vi "DO Test.vi"() -> ()   [LabVIEW 2018]
uses:
  <vilib>/DAQmx/write.llb/DAQmx Write (Digital 1D Bool NChan 1Samp 1Line).vi
  <vilib>/DAQmx/create/channels.llb/DAQmx Create Channel (DO-Digital Output).vi
  <vilib>/DAQmx/miscellaneous.llb/DAQmx Fill In Error Info.vi
  <resource>/objmgr/daqmx.rc
panel:
  in  "index":i32
  out "Array":tag[](array[tag])
  in  "data 2":bool
  in  "Stop":bool
  out "DO.Lines":tag[](array[tag])
  out "DevNames":tag[](array[tag])
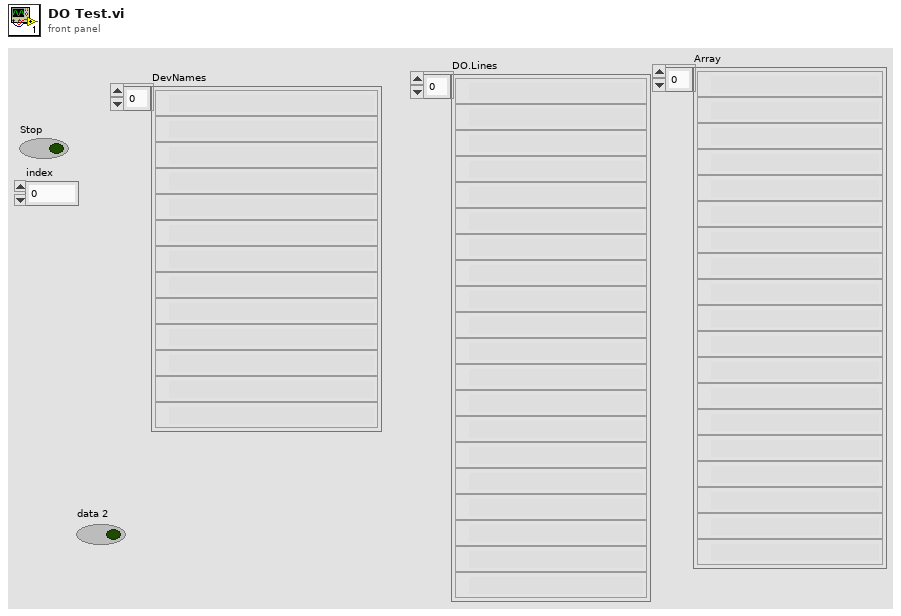
[diagram p1: front panel]
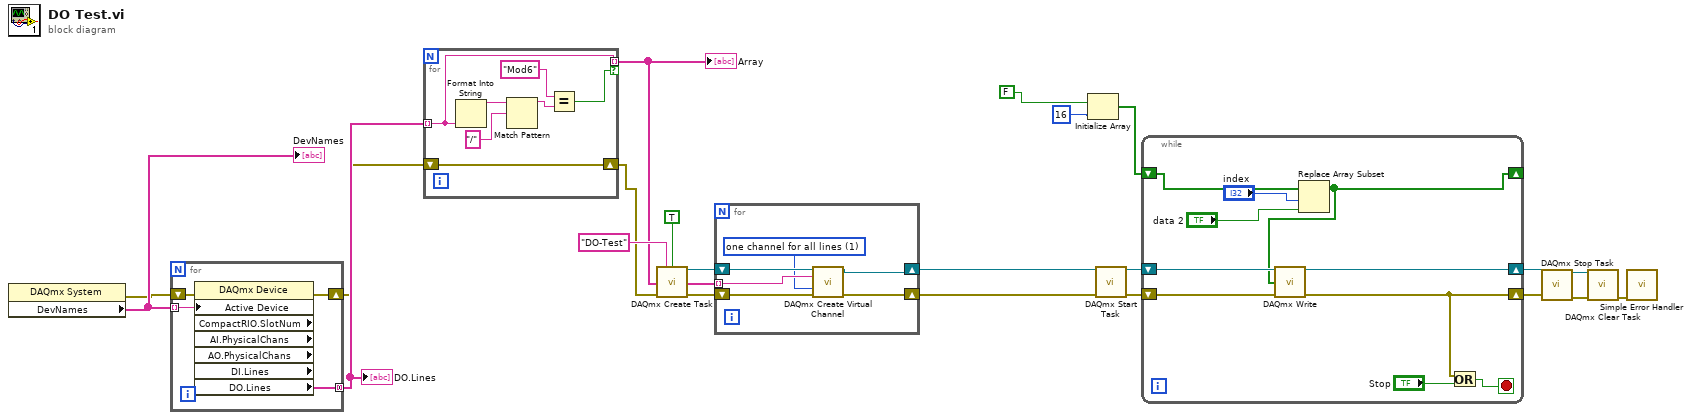
[diagram p0: block diagram]
diagram:
  n1 = property class="DAQmx System"() -> (error out=w17:errorcluster, "DevNames"=w22:tag[])  [unwired: 2 in, 1 out]
  "DevNames" <- w22
  n2 = for {
    tunnel: w22 -> [w26] mode=indexing
    tunnel: [w25] -> w8 mode=concatenating
    shift-right: [w24] -> w6
    shift-left: w17 -> [w23]
    n3 = property class="DAQmx Device" props=["Active Device", "CompactRIO.SlotNum", "AI.PhysicalChans", "AO.PhysicalChans", "DI.Lines", "DO.Lines"](error in=w23, "Active Device"=w26) -> (error out=w24:errorcluster, "DO.Lines"=w25:tag[])  [unwired: 1 in, 5 out]
  }
  "DO.Lines" <- w8
  n4 = for {
    tunnel: w8 -> [w29] mode=indexing
    tunnel: [w29] -> w9 mode=indexing if=w28
    shift-right: [w27] -> w7
    shift-left: w6 -> [w27]
    n5 = Format Into String(w29) -> (resulting string=w33:string)  [unwired: 3 in, 1 out]
    n6 = Match Pattern(string=w33, regular expression="/") -> (before substring=w31:string)  [unwired: 1 in, 3 out]
    n7 = Equal?(x="Mod6" ("before substring"), y=w31) -> (x = y?=w28:bool)
  }
  "Array" <- w9
  n8 = call <vilib>:"DAQmx Create Task.vi"("new task name"="DO-Test", "auto cleanup"=TRUE, "error in"=w7) -> ("task out"=w18:refnum<k21>, "error out"=w19:errorcluster)  [unwired: 11 in]
  n9 = for {
    shift-right: [w37] -> w1
    shift-left: w18 -> [w38]
    tunnel: w9 -> [w36] mode=indexing
    shift-right: [w34] -> w2
    shift-left: w19 -> [w39]
    w35 = 1 items=["one channel for each line", "one channel for all lines"] ("line grouping")
    n10 = call-poly <vilib>:"DAQmx Create Virtual Channel.vi"("task in"=w38, "lines"=w36, "line grouping"=w35, "error in"=w39) -> ("task out"=w37:refnum<k21>, "error out"=w34:errorcluster)  [unwired: 10 in]
  }
  n11 = Initialize Array(FALSE, 16 ("dimension size")) -> (w3:bool[])
  n12 = call <vilib>:"DAQmx Start Task.vi"("task/channels in"=w1, "error in"=w2) -> ("task out"=w16:refnum<k21>, "error out"=w15:errorcluster)  [unwired: 12 in]
  n13 = while {
    shift-right: [w44] -> w11
    shift-left: w16 -> [w49]
    shift-right: [w47] -> w14
    shift-left: w15 -> [w48]
    shift-right: [w42] -> _
    shift-left: w3 -> [w43]
    stop <- w45 stop-if-true
    n14 = Replace Array Subset(array=w43, new element="data 2", index="index") -> (w42:bool[])
    n15 = call-poly <vilib>:"DAQmx Write.vi"("task/channels in"=w49, "data"=w42, "error in"=w48) -> ("task out"=w44:refnum<k21>, "error out"=w47:errorcluster)  [unwired: 10 in, 1 out]
    n16 = Or(x=w47, y="Stop") -> (x .or. y?=w45:bool)
  }
  n17 = call <vilib>:"DAQmx Stop Task.vi"("task/channels in"=w11, "error in"=w14) -> ("task out"=w10:refnum<k21>, "error out"=w13:errorcluster)  [unwired: 12 in]
  n18 = call <vilib>:"DAQmx Clear Task.vi"("task in"=w10, "error in"=w13) -> ("error out"=w12:errorcluster)  [unwired: 13 in]
  n19 = call <vilib>:"Simple Error Handler.vi"("error in (no error)"=w12) -> ()  [unwired: 4 in, 5 out]
